vi "XIPIN_LTE_PUCCH_Receiver_2_0.vi"   [LabVIEW 2017]
doc: "The LTE PUCCH Receiver core provides designers with an LTE Physical Uplink Control Channel Receiver block for the 3GPP TS 36.211 v9.0.0 Physical Channels and Modulation (Release 9) specification. It provides channel estimation, demodulation and decoding.\n------------------------------------\n<b>Need License</b> : Yes\n<b>Interface</b> : AXI4-Stream"
uses:
  <vilib>/rvi/XilinxIP/XIPIN_XNode/niFpgaXIPIN.xnode
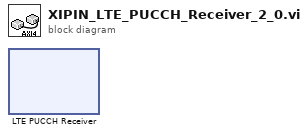
[diagram p0: block diagram]
diagram:
  n1 = xnode ("LTE PUCCH Receiver")() -> ()
